vi "T1T2占空比2.vi"   [LabVIEW 2020]
uses:
  Global_Variable/Global.vi
  <userlib>/DAQNavi Polymorphic VI/create/DAQNavi Create Channel(CI-PulseWidth).vi
  <userlib>/DAQNavi Polymorphic VI/read/DAQNavi Read (Counter Pulse Width 1Chan 1Samp).vi
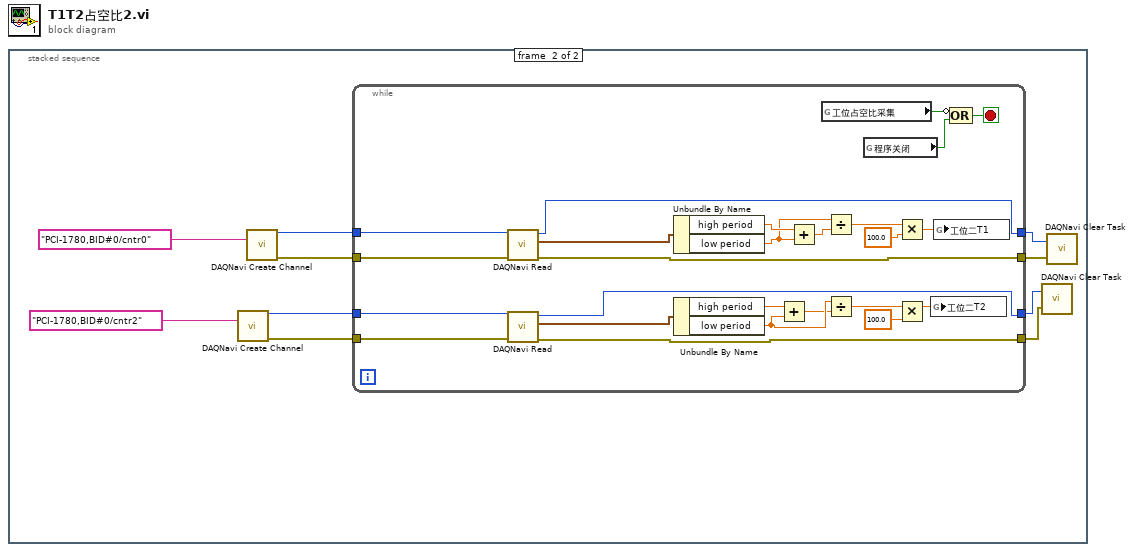
[diagram p0: block diagram]
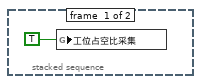
[diagram p2: hidden frame]
diagram:
  n1 = stacked-sequence {
    frame #0 {
      n2 = global write "Global.vi" "工位占空比采集"(TRUE ("工位一占空比采集")) -> ()
    }
    frame #1 {
      n3 = call-poly <userlib>:"DAQNavi Create Channel.vi"("physical channels"="PCI-1780,BID#0/cntr2") -> ("task out"=w4:i32, "error out"=w3:errorcluster)  [unwired: 13 in]
      n4 = call-poly <userlib>:"DAQNavi Create Channel.vi"("physical channels"="PCI-1780,BID#0/cntr0") -> ("task out"=w8:i32, "error out"=w7:errorcluster)  [unwired: 13 in]
      n5 = while {
        tunnel: w8 -> [w27]
        tunnel: [w28] -> w10
        tunnel: w7 -> [w26]
        tunnel: [w29] -> w11
        tunnel: w4 -> [w14]
        tunnel: [w13] -> w5
        tunnel: w3 -> [w15]
        tunnel: [w12] -> w2
        stop <- w30 stop-if-true
        n6 = call-poly <userlib>:"DAQNavi Read.vi"("error in (no error)"=w26, "task in"=w27) -> ("error out"=w29:errorcluster, "data"=w36:cluster{"high period":dbl, "low period":dbl}, "task out"=w28:i32)  [unwired: 7 in]
        n7 = call-poly <userlib>:"DAQNavi Read.vi"("error in (no error)"=w15, "task in"=w14) -> ("error out"=w12:errorcluster, "data"=w18:cluster{"high period":dbl, "low period":dbl}, "task out"=w13:i32)  [unwired: 7 in]
        n8 = Unbundle By Name(w36) -> ("high period"=w24:dbl, "low period"=w23:dbl)
        n9 = Unbundle By Name(w18) -> ("high period"=w21:dbl, "low period"=w22:dbl)
        n10 = Add(x=w21, y=w22) -> (x+y=w19:dbl)
        n11 = Add(x=w24, y=w23) -> (x+y=w35:dbl)
        n12 = global read "Global.vi" "工位占空比采集"() -> (w32:bool)
        n13 = Divide(x=w23, y=w35) -> (x/y=w34:dbl)
        n14 = Divide(x=w22, y=w19) -> (x/y=w20:dbl)
        n15 = global read "Global.vi" "程序关闭"() -> (w31:bool)
        n16 = Multiply(x=w34, y=100.0) -> (x*y=w25:dbl)
        n17 = Multiply(x=w20, y=100.0) -> (x*y=w17:dbl)
        n18 = global write "Global.vi" "工位二T2"(w17) -> ()
        n19 = global write "Global.vi" "工位二T1"(w25) -> ()
        n20 = Compound Arithmetic op=OR ("复合运算")(invert w32, w31) -> (w30:bool)
      }
      n21 = call <userlib>:"DAQNavi Clear Task.vi"("error in (no error)"=w2, "task in"=w5) -> ()  [unwired: 1 in, 1 out]
      n22 = call <userlib>:"DAQNavi Clear Task.vi"("error in (no error)"=w11, "task in"=w10) -> ()  [unwired: 1 in, 1 out]
    }
  }
